vi "get_price.vi"(8 "error in (no error)":errorcluster, 11 "ChairWithTableAttached in":refnum<class "ChairWithTableAttached.lvclass">) -> (0 "error out":errorcluster, 2 "price":dbl, 3 "ChairWithTableAttached out":refnum<class "ChairWithTableAttached.lvclass">)   [LabVIEW 2021, in "ChairWithTableAttached.lvclass"]
uses:
  ChairWithTableAttached.lvclass
  ChairWithTableAttached.lvclass/ChairWithTableAttached.ctl
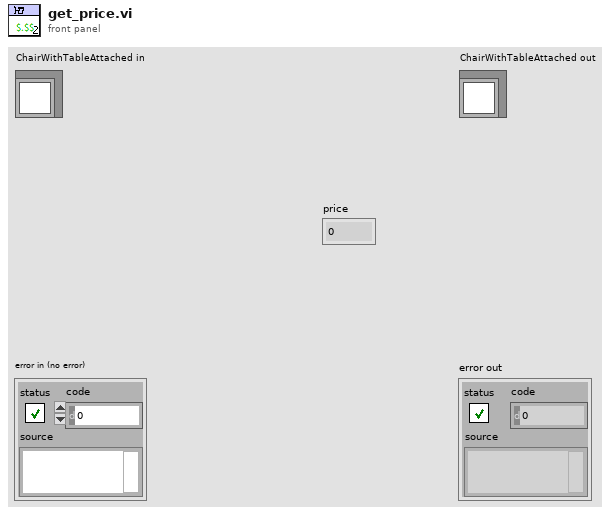
[diagram p1: front panel]
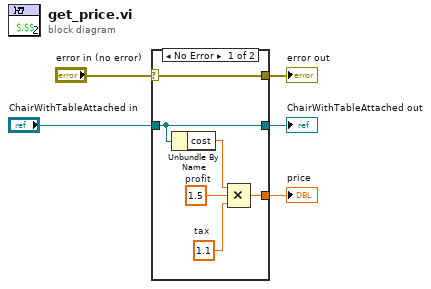
[diagram p0: block diagram]
diagram:
  n1 = case shown="No Error" "error in (no error)" {
    selector: "error in (no error)" -> [w11 w13]
    tunnel: [w11 w13] -> w2
    tunnel: [w10 w12] -> w4
    tunnel: "ChairWithTableAttached in" -> [w10 w12]
    tunnel: [w6 _] -> w1
    frame No Error {
      w7 = 1.1  # tax
      w8 = 1.5  # profit
      n2 = Unbundle By Name(w10) -> ("cost"=w9:dbl)
      n3 = Compound Arithmetic op=MULTIPLY(w9, w8, w7) -> (w6:dbl)
    }
    frame Error {
    }
  }
  "error out" <- w2
  "ChairWithTableAttached out" <- w4
  "price" <- w1
